vi "User_Event_FGV.vi"(8 "error in (no error)":errorcluster, 11 "Enum":T1) -> (0 "error out":errorcluster, 3 "User Event out":refnum<user-event>)   [LabVIEW 2024, in "PCANusb_DTU.lvlib"]
doc: "This VI\n-----------------------------------------------------\nUesr Event FGV\n-----------------------------------------------------\n-Create a user events reference.\n-events can be register with different modules."
uses:
  PCANusb_DTU.lvlib
  Controls/User_Events_Action_Control.ctl
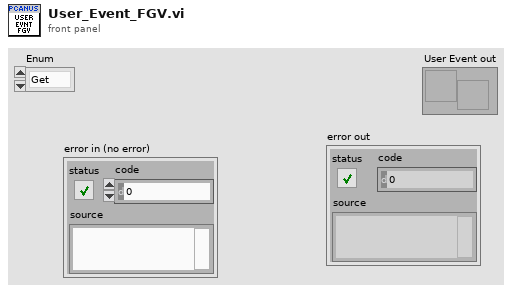
[diagram p1: front panel]
types:
  T1 = typedef "PCANusb_DTU.lvlib/User_Events_Action_Control.ctl" = enum16{"Get", "Create", "Destroy"}
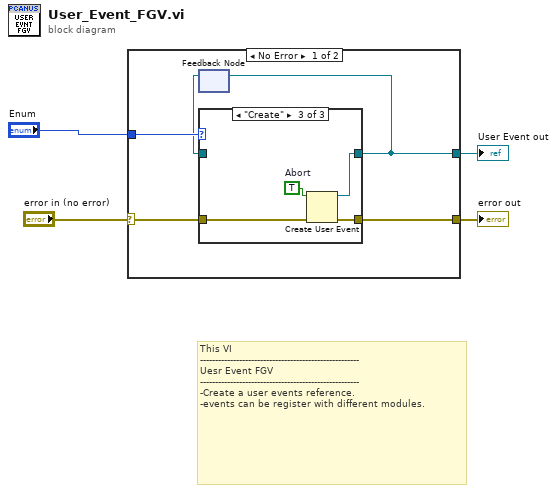
[diagram p0: block diagram]
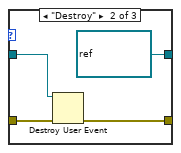
[diagram p3: hidden frame]
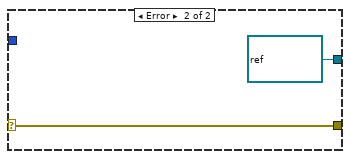
[diagram p4: hidden frame]
diagram:
  # "This VI\n-----------------------------------------------------\nUesr Event FGV\n-----------------------------------------------------\n-Create a user events reference.\n-events can be register with different modules."
  n1 = case shown="No Error" "error in (no error)" {
    selector: "error in (no error)" -> [w9 w21]
    tunnel: [w8 w21] -> w2
    tunnel: [w6 refnum<user-event> refnum ("user event")] -> w3
    tunnel: "Enum" -> [w7 _]
    frame No Error {
      n2 = feedback #1() -> (w5:refnum<user-event>)  [unwired: 1 in]
      n3 = case shown="\"Create\"" w7 {
        tunnel: w9 -> [w10 w15 w19]
        tunnel: [w10 w14 w18] -> w8
        tunnel: [w11 refnum<user-event> refnum ("user event") w17] -> w6
        tunnel: w5 -> [w11 w13 _]
        frame "Get", Default {
        }
        frame "Destroy" {
          n4 = Destroy User Event(user event=w13, error in=w15) -> (error out=w14:errorcluster)
        }
        frame "Create" {
          w16 = TRUE  # Abort
          n5 = Create User Event(user event datatype=w16, error in=w19) -> (user event=w17:refnum<user-event>, error out=w18:errorcluster)
        }
      }
      n6 = feedback-in #1(w6) -> ()
    }
    frame Error {
    }
  }
  "User Event out" <- w3
  "error out" <- w2
